vi "Untitled 2.vi"() -> ()   [LabVIEW 2018]
uses:
  vis/Private/Put_DBL-1D_PV-1D.vi
panel:
  in  "stop":bool
  in  "Numeric":dbl format="%#_13g"
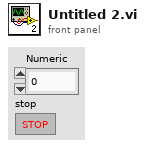
[diagram p1: front panel]
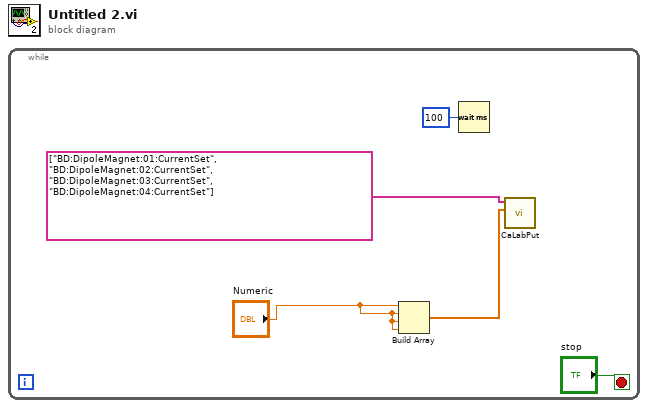
[diagram p0: block diagram]
diagram:
  n1 = while {
    stop <- "stop" stop-if-true
    n2 = Build Array("Numeric", "Numeric", "Numeric", "Numeric") -> (w3:dbl[])
    n3 = Wait (ms)(milliseconds to wait=u32 100) -> ()  [unwired: 1 out]
    n4 = call-poly "CaLabPut.vi"("Values"=w3, "PV Names"=string[] ["BD:DipoleMagnet:01:CurrentSet", "BD:DipoleMagnet:02:CurrentSet", "BD:DipoleMagnet:03:CurrentSet", "BD:DipoleMagnet:04:CurrentSet"]) -> ()  [unwired: 6 in, 4 out]
  }
